vi "rs3 query devices2.vi"(8 "error in (no error)":errorcluster, 11 "rscontext":u64) -> (0 "error out":errorcluster, 1 "error":u64, 3 "device_list":u64)   [LabVIEW 2023]
doc: "Creates a list of devices connected to the PC\n\nINPUT: \nContext This handle in received from INIT API\n\nOUTPUT: \nDevice list Handle to the array of devices\nError 0=no error"
panel:
  # "RS3 Query Devices"
  # "(C) Intel Corp.,  AGJ"
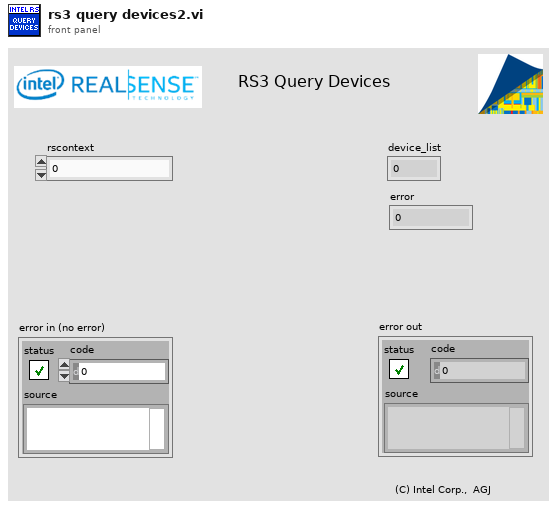
[diagram p1: front panel]
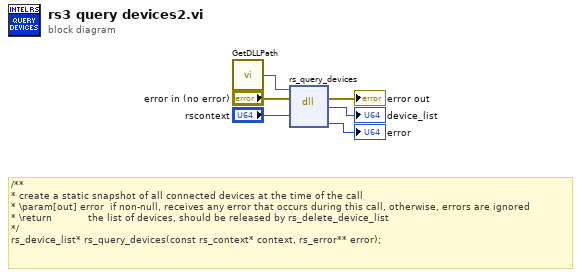
[diagram p0: block diagram]
diagram:
  # "/**\n* create a static snapshot of all connected devices at the time of the call\n* \\param[out] error  if non-null, receives any error that occurs during this call, otherwise, errors are ignored\n* \\return            the list of devices, should be released by rs_delete_device_list\n*/\nrs_device_list* rs_query_devices(const rs_context* context, rs_error** error);"
  n1 = call "GetDLLPath.vi"() -> ("DLL Path"=w1:path)
  n2 = dll-call lib="C:/STEAMSyndicate/RealSenseWrappers/VI Wrappers (add ons) Public/RealSense/realsense-d.dll" fn="rs_query_devices"(path in=w1, error in="error in (no error)", "rscontext"="rscontext") -> (error out=→"error out":errorcluster, "device_list"=→"device_list":u32, "error"=→"error":u64)  [unwired: 3 in, 1 out]
